vi "SubVI_Remove.vi"(10 "Kullanıcı Listesi in":T1, 11 "Silinecek ID":dbl) -> (3 "Kullanıcı Listesi out":T1)   [LabVIEW 2024]
uses:
  Control 3.ctl
  Documents/LabView Projects/Control 1.ctl
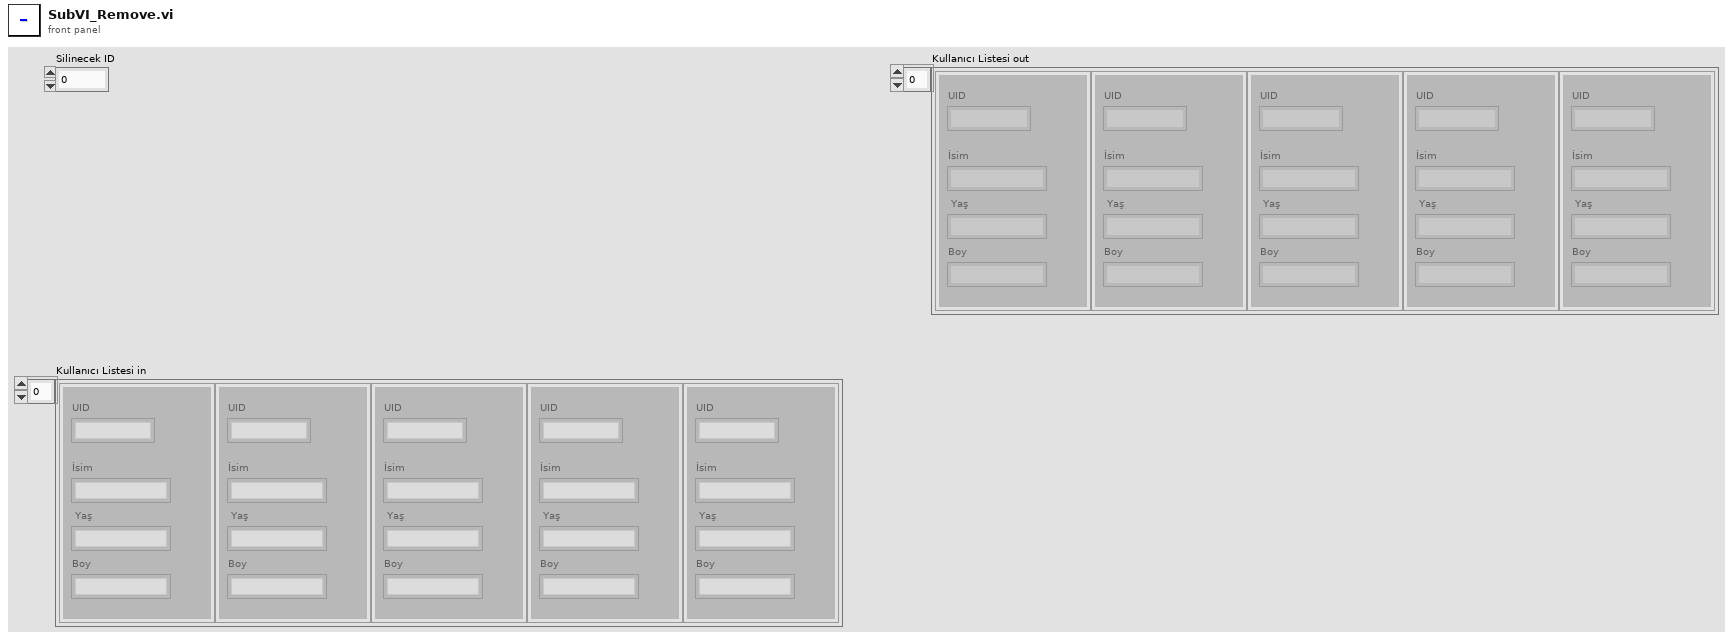
[diagram p1: front panel]
types:
  T1 = typedef "Control 3.ctl" = T2[]
  T2 = typedef "Control 1.ctl" = cluster{"UID":string, "İsim":string, " Yaş":string, "Boy":string}
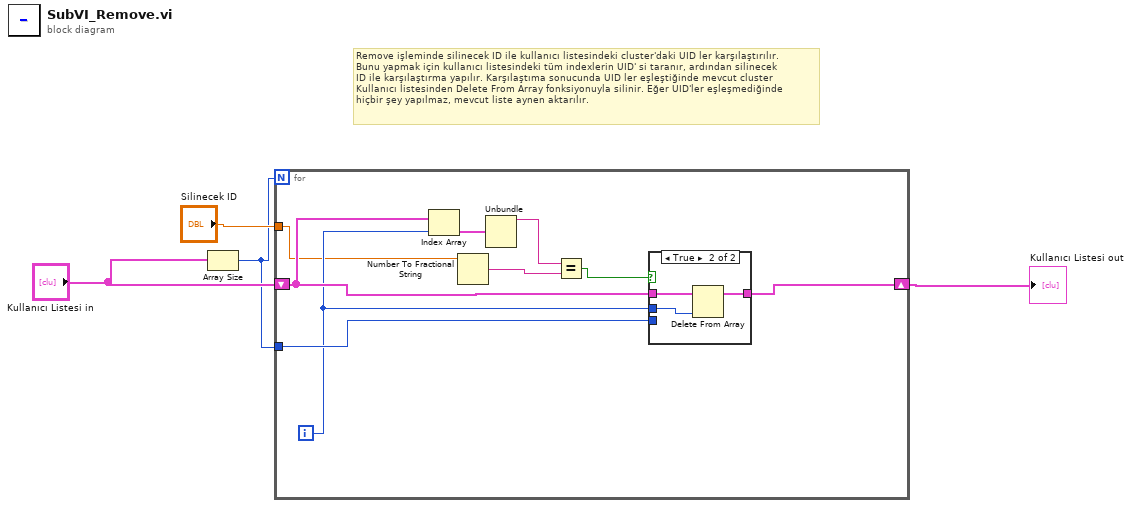
[diagram p0: block diagram]
diagram:
  # "Remove işleminde silinecek ID ile kullanıcı listesindeki cluster'daki UID ler karşılaştırılır.\nBunu yapmak için kullanıcı listesindeki tüm indexlerin UID' si taranır, ardından silinecek\nID ile karşılaştırma yapılır. Karşılaştıma sonucunda UID ler eşleştiğinde mevcut cluster \nKullanıcı listesinden Delete From Array fonksiyonuyla silinir. Eğer UID'ler eşleşmediğinde\nhiçbir şey yapılmaz, mevcut liste aynen aktarılır."
  n1 = Array Size(array="Kullanıcı Listesi in") -> (size(s)=w1:i32)
  n2 = for {
    N: w1 -> [_]
    tunnel: w1 -> [w10]
    shift-right: [w7] -> w4
    shift-left: "Kullanıcı Listesi in" -> [w9]
    tunnel: "Silinecek ID" -> [w6]
    i -> [w8]
    n3 = Index Array(array=w9, index=w8) -> (element=w13:T2)
    n4 = Number To Fractional String(number=w6) -> (F-format string=w5:string)  [unwired: 3 in]
    n5 = Unbundle(w13) -> ("UID"=w12:string)  [unwired: 3 out]
    n6 = Equal?(x=w12, y=w5) -> (x = y?=w11:bool)
    n7 = case shown="True" w11 {
      tunnel: w10 -> [_ _]
      tunnel: w9 -> [w14 w17]
      tunnel: w8 -> [_ w16]
      tunnel: [w14 w15] -> w7
      frame False {
      }
      frame True {
        n8 = Delete From Array(array=w17, index=w16) -> (array with subset deleted=w15:T1)  [unwired: 1 in, 1 out]
      }
    }
  }
  "Kullanıcı Listesi out" <- w4
